vi "Generate File Name.vi"(10 "name or relative path":string="Test.tif", 11 "base path":path=path "C:/Users/BoasLab/Documents/Data/Alazar data/B-line") -> (3 "appended path":path)   [LabVIEW 2018]
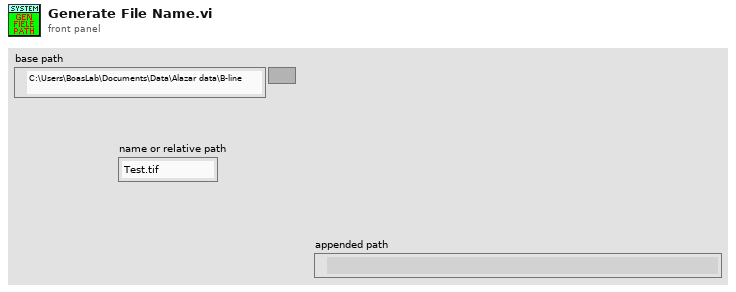
[diagram p1: front panel]
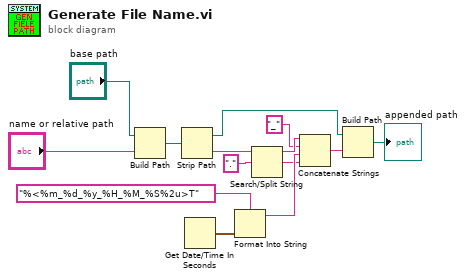
[diagram p0: block diagram]
diagram:
  n1 = Build Path(base path="base path", name or relative path="name or relative path") -> (appended path=w7:path)
  n2 = Strip Path(path=w7) -> (stripped path=w10:path, name=w14:string)
  n3 = Get Date/Time In Seconds() -> (seconds since 1Jan1904=w6:timestamp)
  n4 = Format Into String(format string="%<%m_%d_%y_%H_%M_%S%2u>T", w6) -> (resulting string=w4:string)  [unwired: 2 in, 1 out]
  n5 = Search/Split String(string=w14, search string/char (-)=".") -> (substring before match=w12:string, match + rest of string=w1:string)  [unwired: 1 in, 1 out]
  n6 = Concatenate Strings(w12, "_" ("string"), w4, w1) -> (w11:string)
  n7 = Build Path(base path=w10, name or relative path=w11) -> (appended path=→"appended path":path)
